vi "ColorScale.vi"(8 "error in (no error)":errorcluster, 10 "ColorScale Label":string, 11 "ITX Commands in":refnum<class "ITX Commands.lvclass">) -> (0 "error out":errorcluster, 3 "ITX Commands out":refnum<class "ITX Commands.lvclass">)   [LabVIEW 2019, in "ITX Commands.lvclass"]
uses:
  ITX Commands.lvclass
  ITX Commands.lvclass/ITX Commands.ctl
panel:
  out "resulting string":string="ModifyImage '' ctab{,, Rainbow, 0}"
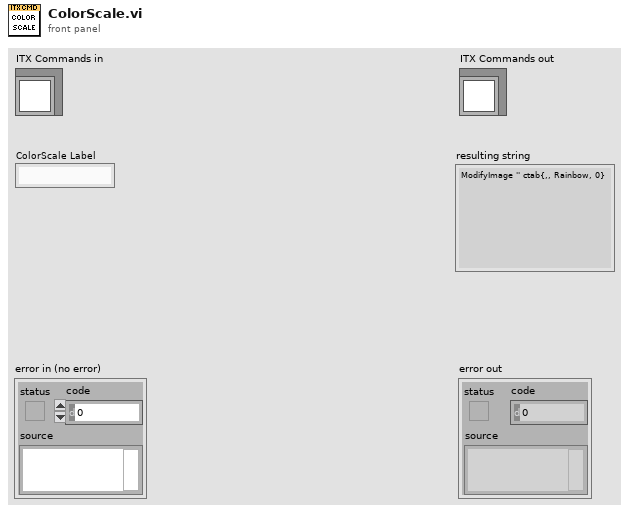
[diagram p1: front panel]
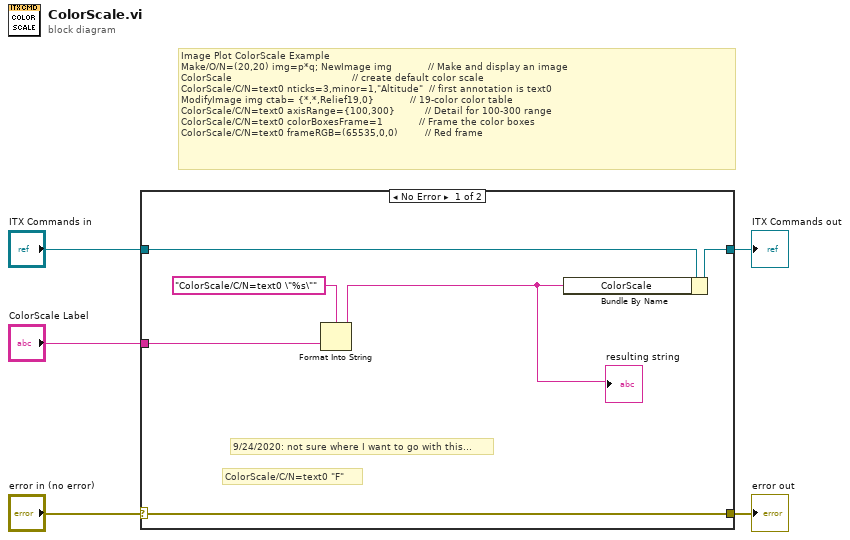
[diagram p0: block diagram]
diagram:
  # "Image Plot ColorScale Example\nMake/O/N=(20,20) img=p*q; NewImage img\t\t\t         // Make and display an image\nColorScale\t\t\t\t\t\t                                  // create default color scale\nColorScale/C/N=text0 nticks=3,minor=1,\"Altitude\"\t // first annotation is text0\nModifyImage img ctab= {*,*,Relief19,0}\t\t\t         // 19-color color table\nColorScale/C/N=text0 axisRange={100,300}\t\t        // Detail for 100-300 range\nColorScale/C/N=text0 colorBoxesFrame=1\t\t\t         // Frame the color boxes\nColorScale/C/N=text0 frameRGB=(65535,0,0)\t\t       // Red frame"
  n1 = case shown="No Error" "error in (no error)" {
    selector: "error in (no error)" -> [w9 w13]
    tunnel: [w9 w13] -> w4
    tunnel: [w10 w12] -> w2
    tunnel: "ITX Commands in" -> [w11 w12]
    tunnel: "ColorScale Label" -> [w8 _]
    frame No Error {
      # "ColorScale/C/N=text0 \"F\""
      # "9/24/2020: not sure where I want to go with this..."
      n2 = Format Into String(format string="ColorScale/C/N=text0 \"%s\"", w8) -> (resulting string=w6:string)  [unwired: 2 in, 1 out]
      "resulting string" <- w6
      n3 = Bundle By Name(cluster=w11, "ColorScale"=w6) -> (w10:refnum<class "ITX Commands.lvclass">)
    }
    frame Error {
    }
  }
  "error out" <- w4
  "ITX Commands out" <- w2
